vi "parseDataU32.vi"(8 "error in (no error)":errorcluster, 11 "FrameParser in":refnum<class "DynamicFrameParser.lvclass">) -> (0 "error out":errorcluster, 2 "Data":u32, 3 "FrameParser out":refnum<class "DynamicFrameParser.lvclass">)   [LabVIEW 2016, in "DynamicFrameParser.lvclass"]
uses:
  DynamicFrameParser.lvclass
  DynamicFrameParser.lvclass/DynamicFrameParser.ctl
  Common_RT_Utilities/U8ArrayParser/U8ArrayParserManualIndexing.lvclass
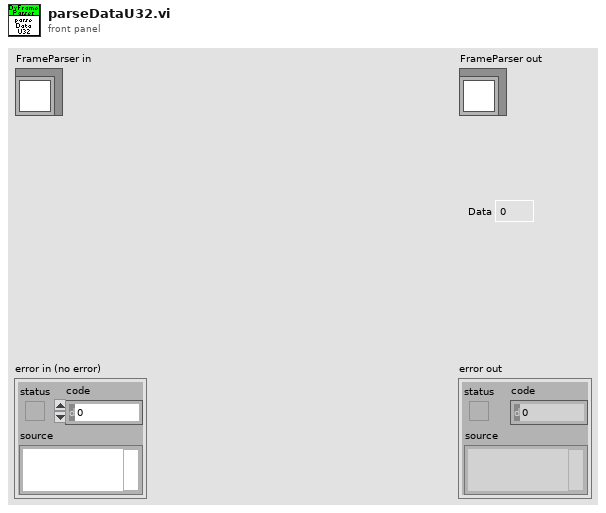
[diagram p1: front panel]
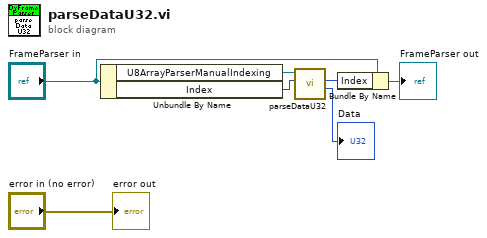
[diagram p0: block diagram]
diagram:
  n1 = Unbundle By Name("FrameParser in") -> ("U8ArrayParserManualIndexing"=w5:refnum<class "U8ArrayParserManualIndexing.lvclass">, "Index"=w4:i32)
  n2 = call "parseDataU32.vi"("Index"=w4, "U8ArrayParserManualIndexing in"=w5) -> ("Data"=→"Data":u32, "Index out"=w3:i32)  [unwired: 6 in, 2 out]
  n3 = Bundle By Name(cluster="FrameParser in", "Index"=w3) -> (→"FrameParser out":refnum<class "DynamicFrameParser.lvclass">)
  "error out" <- "error in (no error)"
